vi "AalborgDFCConfigure.vi"(0 "Address":u8, 1 "Port Name":string, 2 "ConfigString":string, 3 "Channel Name":string) -> (8 "Good Echo":bool)   [LabVIEW 2021]
panel:
  out "Array 2":string[](array[string])
  out "Array":bool[](array[boolean])
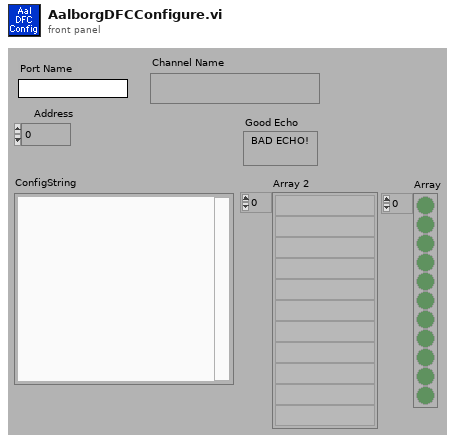
[diagram p1: front panel]
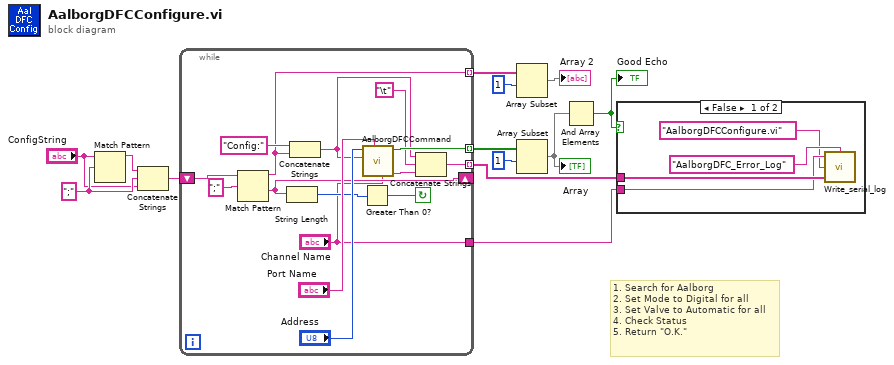
[diagram p0: block diagram]
diagram:
  w11 = ";" ("regular expression")
  # "1. Search for Aalborg\n2. Set Mode to Digital for all\n3. Set Valve to Automatic for all\n4. Check Status\n5. Return \"O.K.\""
  n1 = Match Pattern(string="ConfigString", regular expression=w11) -> (before substring=w12:string)  [unwired: 4 out]
  n2 = Concatenate Strings(w12, w11, "ConfigString") -> (w13:string)
  n3 = while {
    shift-right: [w21] -> _
    shift-left: w13 -> [w26]
    tunnel: [w20] -> w10 mode=indexing
    tunnel: [w19] -> w6 mode=indexing
    tunnel: [w15] -> w3 mode=indexing
    tunnel: ["Channel Name"] -> w2
    stop <- w23 continue-if-true
    n4 = Match Pattern(string=w26, regular expression=";") -> (before substring=w19:string, after substring=w21:string)  [unwired: 3 out]
    n5 = String Length(string=w21) -> (length=w22:i32)
    n6 = Concatenate Strings("Config:" ("string"), w19) -> (w18:string)
    n7 = Greater Than 0?(x=w22) -> (x > 0?=w23:bool)
    n8 = call "AalborgDFCCommand.vi"("Channel Name"="Channel Name", "Port Name"="Port Name", "AalborgDFCCommand"=w18, "Address"="Address") -> ("String Reply"=w16:string, "OK"=w20:bool)  [unwired: 2 in, 3 out]
    n9 = Concatenate Strings(w18, "\t", w16) -> (w15:string)
  }
  n10 = Array Subset(array=w6, index=1) -> (→"Array 2":string[])  [unwired: 1 in]
  n11 = Array Subset(array=w10, index=1) -> (w8:bool[])  [unwired: 1 in]
  "Array" <- w8
  n12 = And Array Elements(Boolean array=w8) -> (logical AND=w1:bool)
  "Good Echo" <- w1
  n13 = case shown="False" w1 {
    tunnel: w3 -> [w31 _]
    tunnel: w2 -> [w30 _]
    frame False {
      n14 = call "Write_serial_log.vi"("Log Type"="AalborgDFC_Error_Log", "Log Array"=w31, "Header message"="AalborgDFCConfigure.vi", "Channel Name"=w30) -> ()  [unwired: 1 out]
    }
    frame True {
    }
  }
